vi "WT-Voltage-Controller.vi"() -> ()   [LabVIEW 2017]
uses:
  <vilib>/Platform/TimedLoop/XDataNode/timing_clust.ctl
  <vilib>/Platform/TimedLoop/XDataNode/nitl_modes.ctl
  <vilib>/Platform/TimedLoop/XDataNode/wakeup.ctl
  <vilib>/platform/TimedLoop/XDataNode/XDataNode.xnode
  <vilib>/Platform/TimedLoop/XDataNode/XDNodeRunTimeDep.lvlib
panel:
  out "Boolean":bool
  in  "POWER":bool
  in  "Sync":bool
  out "error out":errorcluster
  out "Fan 1 Indicator":dbl
  out "Fan 2 Indicator":dbl
  in  "Fan 2 Voltage":dbl(knob) scale=0.0..10.0
  in  "Fan 1 Voltage":dbl(knob) scale=0.0..10.0
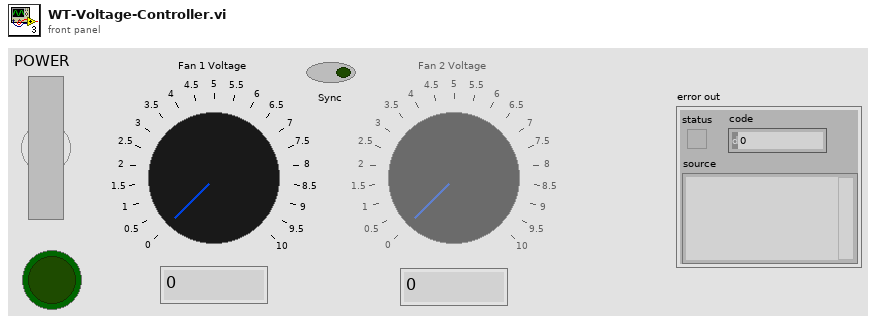
[diagram p1: front panel]
types:
  T1 = typedef "XDNodeRunTimeDep.lvlib/timing_clust.ctl" = cluster{"Expected End [f-1]":u64, "Actual End [f-1]":u64, "Finished Late? [f-1]":bool, "Expected End [i-1]":u64, "Actual End [i-1]":u64, "Finished Late? [i-1]":bool, "Expected Start [i]":u64, "Actual Start [i]":u64, "Expected Start [f]":u64, "Actual Start [f]":u64, "Source Name":string, "Structure Name":string, "Period":i64, "Deadline":i64, "Offset":i64, "Start":i64, "Priority":i32, "Timeout":i32, "Mode":T2, "Wakeup Reason":T3, "Error":errorcluster, "Source Type":string, "Secondary Source Type":string, "Global End Time":u64, "Global Start Time":u64, "Frame Duration":u64, "Iteration Duration":u64, "Assigned CPU":i32, "I/O Scan Engine Mode":u32}
  T2 = typedef "XDNodeRunTimeDep.lvlib/nitl_modes.ctl" = enum32{"No Change", "Process missed periods, maintain original phase", "Discard missed periods, maintain original phase", "Process missed periods, ignore original phase", "Discard missed periods, ignore original phase"}
  T3 = typedef "XDNodeRunTimeDep.lvlib/wakeup.ctl" = enum32{"Normal", "Aborted", "Asynchronous wakeup", "Timing source error", "Timed loop error", "Timeout"}
  T4 = enum8{"Enabled", "Disabled", "Disabled and Grayed Out"}
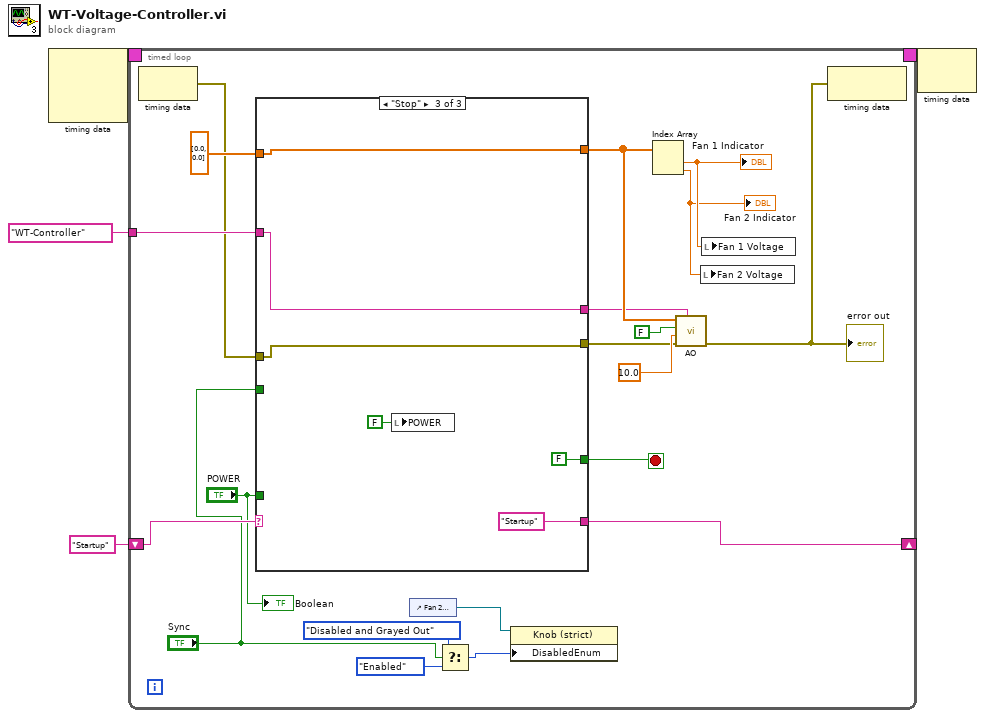
[diagram p0: block diagram]
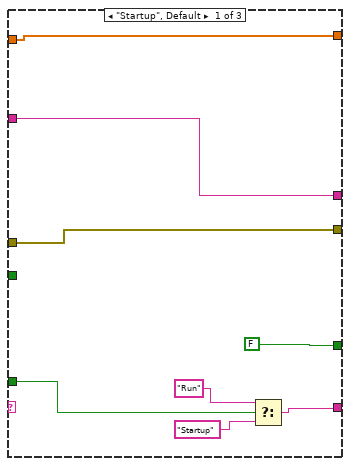
[diagram p2: hidden frame]
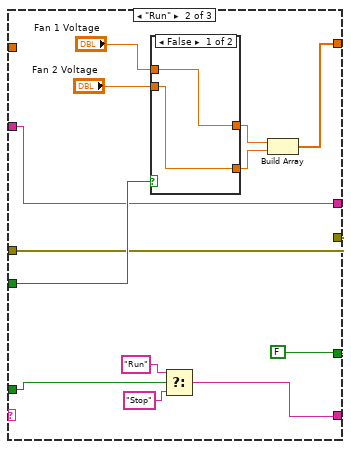
[diagram p3: hidden frame]
diagram:
  n1 = node-c288() -> (w2:T1)  [unwired: 3 in]
  n2 = timed-loop {
    shift-right: [w23] -> _
    shift-left: "Startup" -> [w24]
    tunnel: tag "WT-Controller" ("device name") -> [w21]
    timing: w2 -> [_]
    timing-out: [_] -> w1
    stop <- w22 stop-if-true
    n3 = node-c288() -> (w10:errorcluster)  [unwired: 1 in]
    n4 = case shown="\"Stop\"" w24 {
      tunnel: [w31 w50 "Startup" ("f")] -> w23
      tunnel: [w36 w43 w57] -> w14
      tunnel: [FALSE ("Stop") FALSE ("Stop") FALSE ("Stop")] -> w22
      tunnel: w21 -> [w35 w42 w58]
      tunnel: [w37 w41 w56] -> w12
      tunnel: w10 -> [w37 w41 w56]
      tunnel: "Sync" -> [_ w45 _]
      tunnel: dbl[] [0.0, 0.0] ("appended array") -> [w36 _ w57]
      tunnel: [w35 w42 w58] -> w11
      tunnel: "POWER" -> [w33 w40 _]
      frame "Startup", Default {
        n5 = Select(t="Run" ("f"), s=w33, f="Startup") -> (s? t:f=w31:string)
      }
      frame "Run" {
        n6 = case shown="False" w45 {
          tunnel: [w51 w53] -> w48
          tunnel: [w52 w53] -> w47
          tunnel: "Fan 1 Voltage" -> [w52 w53]
          tunnel: "Fan 2 Voltage" -> [w51 _]
          frame False {
          }
          frame True {
          }
        }
        n7 = Select(t="Run" ("f"), s=w40, f="Stop") -> (s? t:f=w50:string)
        n8 = Build Array(w47, w48) -> (w43:dbl[])
      }
      frame "Stop" {
        n9 = local write "POWER"(FALSE ("POWER")) -> ()
      }
    }
    n10 = control-ref of="Fan 2 Voltage"() -> (w17:refnum<vi>)
    n11 = Select(t=T4."Disabled and Grayed Out" ("Disabled"), s="Sync", f=T4."Enabled") -> (s? t:f=w19:T4)
    n12 = property class="Knob (strict)"(reference=w17, "DisabledEnum"=w19) -> ()  [unwired: 1 in, 2 out]
    n13 = Index Array(array=w14) -> (element #1=w8:dbl, element #2=w7:dbl)  [unwired: 2 in]
    "Fan 1 Indicator" <- w8
    "Fan 2 Indicator" <- w7
    n14 = call "AO.vi"("device name"=w11, "error in"=w12, "timeout (s)"=10.0, "stop (T)"=FALSE, "data"=w14) -> ("error out"=w9:errorcluster)  [unwired: 2 in, 1 out]
    "error out" <- w9
    n15 = local write "Fan 2 Voltage"(w7) -> ()
    n16 = local write "Fan 1 Voltage"(w8) -> ()
    n17 = node-c288(w9) -> ()  [unwired: 1 out]
    "Boolean" <- "POWER"
  }
  n18 = node-c288(w1) -> ()  [unwired: 1 out]
